vi "AllTogether.vi"() -> ()   [LabVIEW 2022 SP3]
uses:
  <vilib>/DAQmx/read.llb/DAQmx Read (Digital Bool 1Line 1Point).vi
  <vilib>/DAQmx/read.llb/DAQmx Read (Analog 1D DBL NChan 1Samp).vi
  <vilib>/DAQmx/write.llb/DAQmx Write (Digital Bool 1Line 1Point).vi
  <vilib>/DAQmx/create/channels.llb/DAQmx Create Channel (AI-Voltage-Basic).vi
  <vilib>/DAQmx/create/channels.llb/DAQmx Create Channel (DO-Digital Output).vi
  <vilib>/DAQmx/miscellaneous.llb/DAQmx Fill In Error Info.vi
  <vilib>/DAQmx/create/channels.llb/DAQmx Create Channel (DI-Digital Input).vi
panel:
  in  "Numeric 3":dbl
  out "error out":errorcluster
  in  "lines 2":tag
  in  "Connect":bool
  in  "VISA resource name":refnum<visa-resource-name>
  out "connected":bool
  in  "Numeric 2":dbl
  in  "stop 3":bool
  out "Weight Range":dbl(knob) scale=0.0..1500.0
  in  "physical channels":tag
  out "Timer":i32
  out "Numeric":i32
  in  "stop":bool
  out "Buzzer":bool
  in  "lines":tag
  # "Smart Refridgerator System"
  # "Weight Sensor"
  # "Contact Sensor"
  # "Water Level sensor and DC motor control"
  # "g"
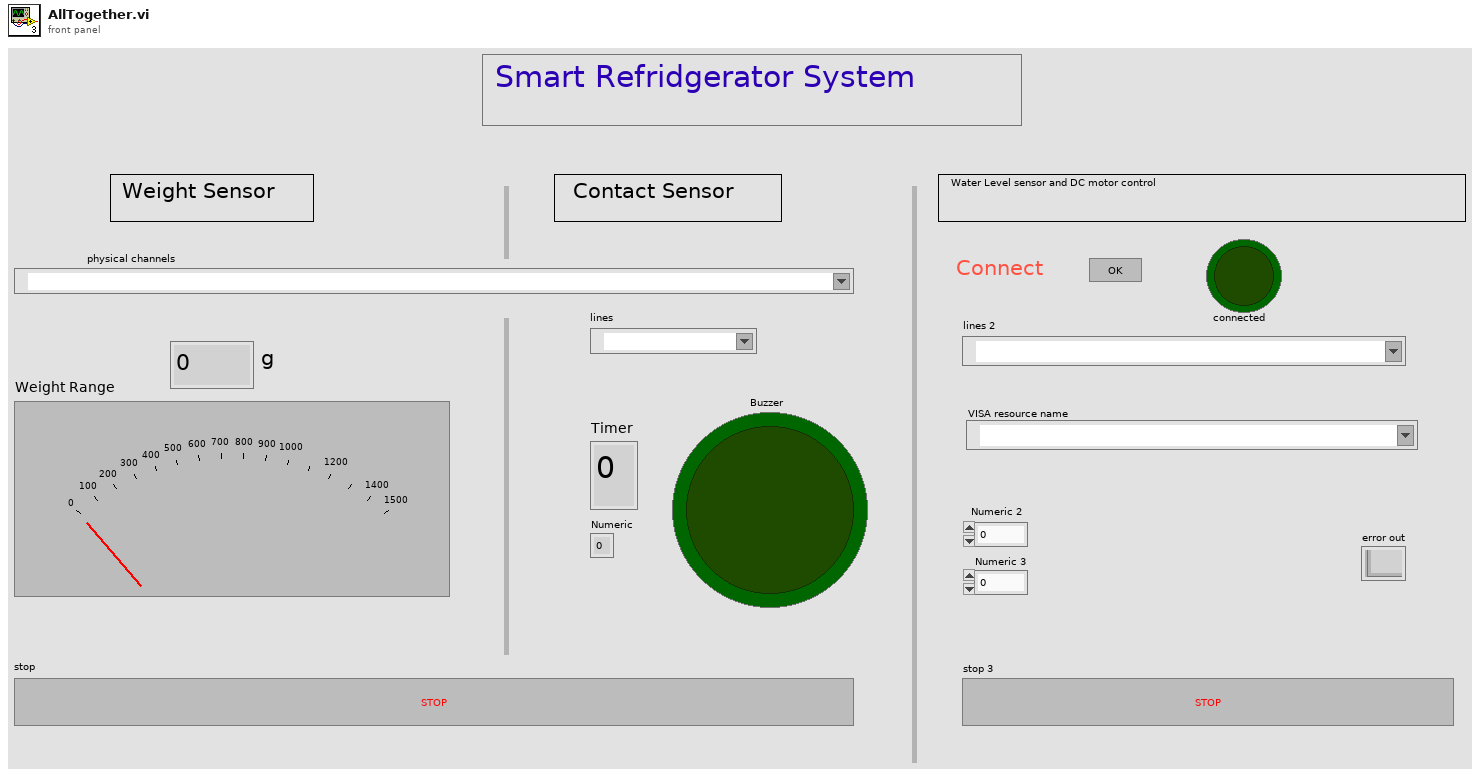
[diagram p1: front panel]
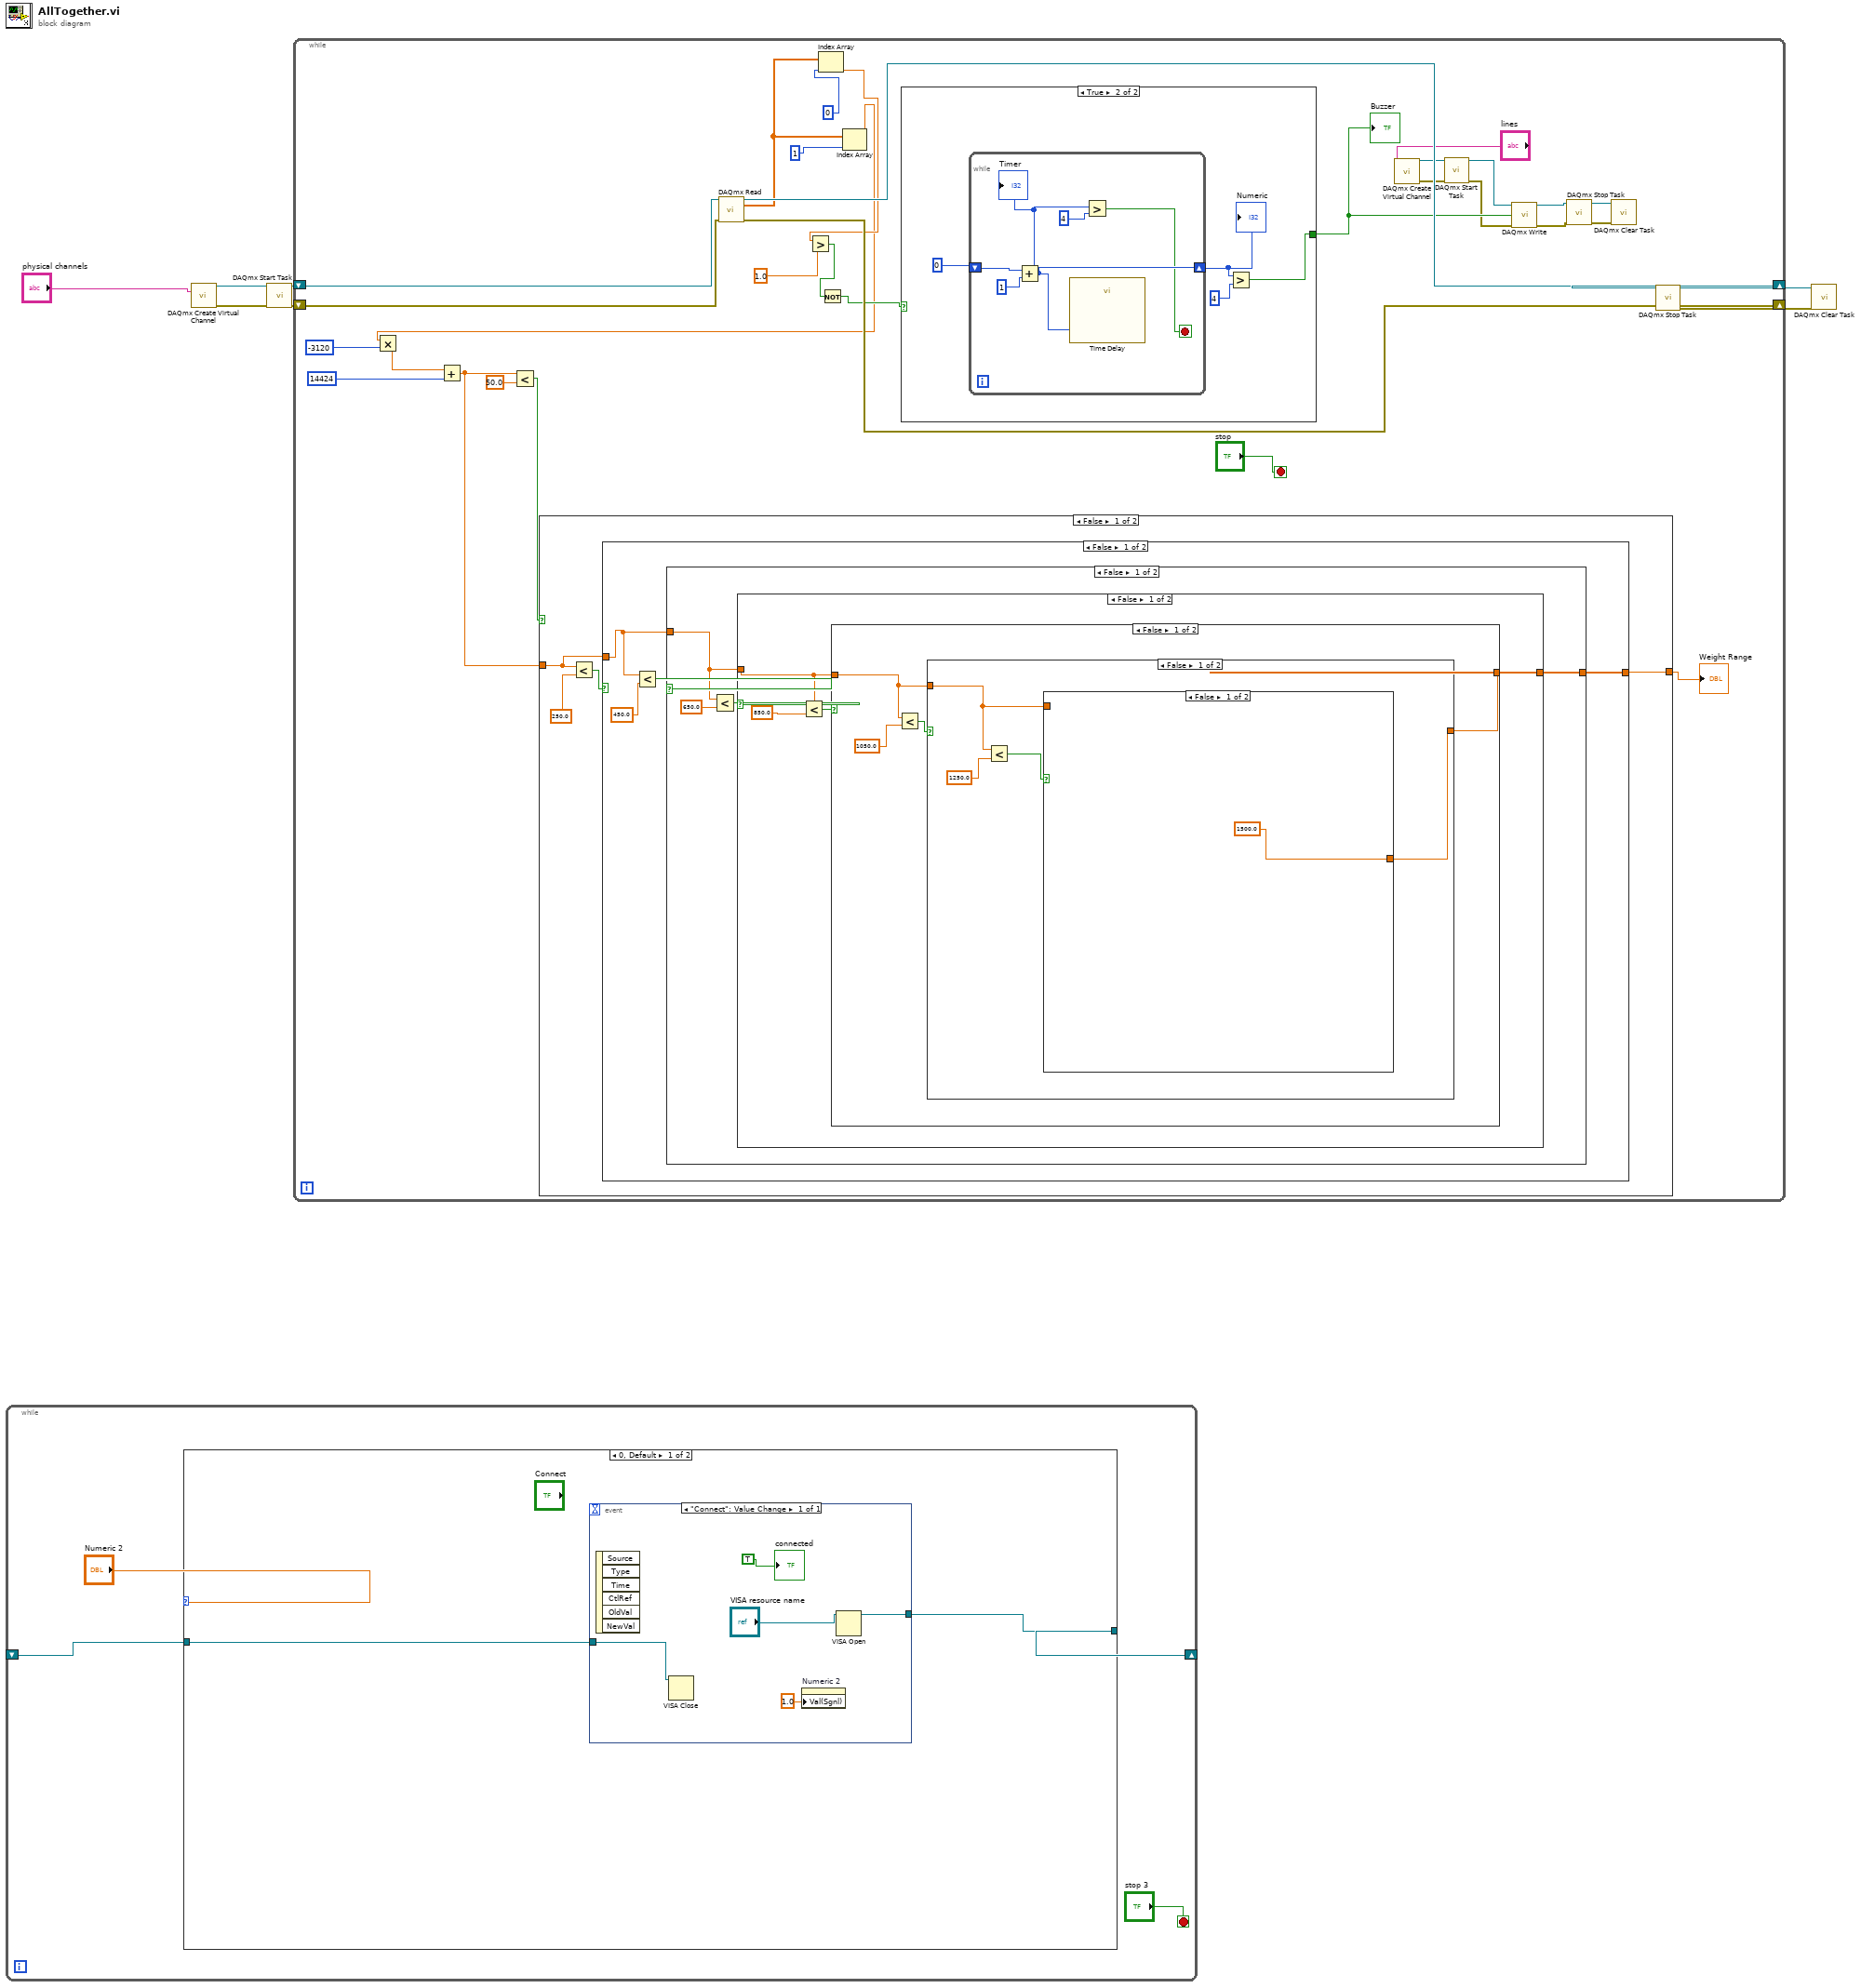
[diagram p0: block diagram]
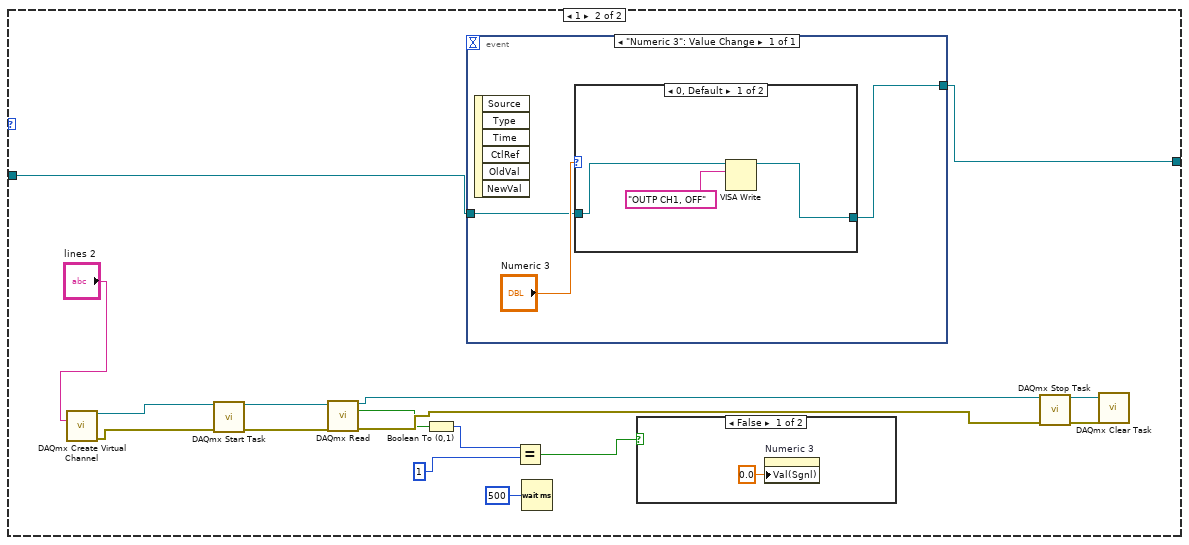
[diagram p2: hidden frame]
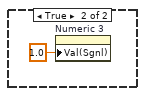
[diagram p3: hidden frame]
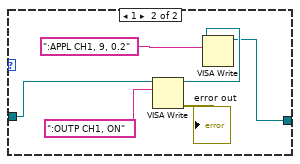
[diagram p4: hidden frame]
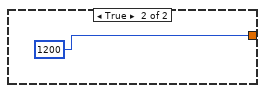
[diagram p5: hidden frame]
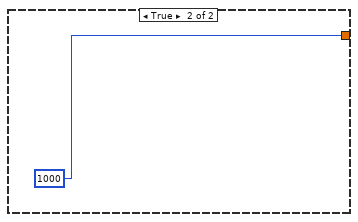
[diagram p6: hidden frame]
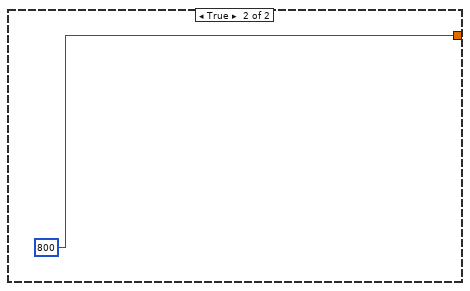
[diagram p7: hidden frame]
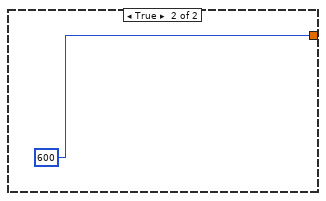
[diagram p8: hidden frame]
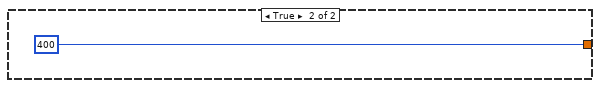
[diagram p9: hidden frame]
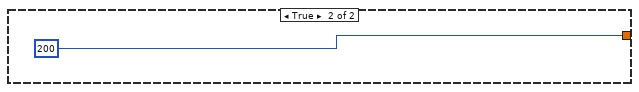
[diagram p10: hidden frame]
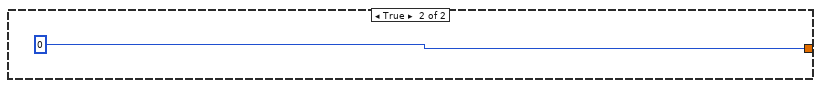
[diagram p11: hidden frame]
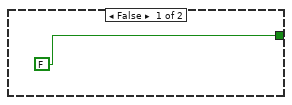
[diagram p12: hidden frame]
diagram:
  n1 = while {
    shift-right: [w13] -> _
    shift-left: _ -> [w11]
    stop <- "stop 3" stop-if-true
    n2 = case shown="0, Default" "Numeric 2" {
      tunnel: [w14 w36] -> w13
      tunnel: w11 -> [w15 w35]
      frame 0, Default {
        n3 = event shown="[0] \"Connect\": Value Change" {
          selector: _ -> [_]
          dyn-events: _ -> [_]
          timeout: _ -> [_]
          tunnel: w15 -> [w20]
          tunnel: [w18] -> w14
          event "Connect": Value Change {
            n4 = event-data() -> ()  [unwired: 1 in, 6 out]
            n5 = VISA Close(VISA resource name=w20) -> ()  [unwired: 1 in, 1 out]
            n6 = property on="Numeric 2" class="DigNum (strict)"("Val(Sgnl)"=1.0 ("Value (Signaling)")) -> ()  [unwired: 2 in, 2 out]
            n7 = VISA Open(VISA resource name="VISA resource name") -> (VISA resource name=w18:refnum<visa-resource-name>)  [unwired: 4 in, 1 out]
            "connected" <- TRUE
          }
        }
      }
      frame 1 {
        n8 = call-poly <vilib>:"DAQmx Create Virtual Channel.vi"("lines"="lines 2") -> ("task out"=w29:refnum<k21>, "error out"=w28:errorcluster)  [unwired: 13 in]
        n9 = call <vilib>:"DAQmx Start Task.vi"("task/channels in"=w29, "error in"=w28) -> ("task out"=w31:refnum<k21>, "error out"=w30:errorcluster)  [unwired: 12 in]
        n10 = call-poly <vilib>:"DAQmx Read.vi"("task/channels in"=w31, "error in"=w30) -> ("task out"=w26:refnum<k21>, "data"=w21:bool, "error out"=w25:errorcluster)  [unwired: 11 in]
        n11 = Boolean To (0,1)(Boolean=w21) -> (0, 1=w33:i16)
        n12 = event shown="[0] \"Numeric 3\": Value Change" {
          selector: _ -> [_]
          dyn-events: _ -> [_]
          timeout: _ -> [_]
          tunnel: [w41] -> w36
          tunnel: w35 -> [w39]
          event "Numeric 3": Value Change {
            n13 = event-data() -> ()  [unwired: 1 in, 6 out]
            n14 = case shown="0, Default" "Numeric 3" {
              tunnel: [w43 w47] -> w41
              tunnel: w39 -> [w42 w46]
              frame 0, Default {
                n15 = VISA Write(VISA resource name=w42, write buffer="OUTP CH1, OFF") -> (VISA resource name out=w43:refnum<visa-resource-name>)  [unwired: 1 in, 2 out]
              }
              frame 1 {
                n16 = VISA Write(VISA resource name=w46, write buffer=":OUTP CH1, ON") -> (VISA resource name out=w48:refnum<visa-resource-name>, error out=→"error out":errorcluster)  [unwired: 1 in, 1 out]
                n17 = VISA Write(VISA resource name=w48, write buffer=":APPL CH1, 9, 0.2") -> (VISA resource name out=w47:refnum<visa-resource-name>)  [unwired: 1 in, 2 out]
              }
            }
          }
        }
        n18 = Equal?(x=w33, y=1) -> (x = y?=w34:bool)
        n19 = Wait (ms)(milliseconds to wait=u32 500) -> ()  [unwired: 1 out]
        n20 = case shown="False" w34 {
          frame False {
            n21 = property on="Numeric 3" class="DigNum (strict)"("Val(Sgnl)"=0.0 ("Value (Signaling)")) -> ()  [unwired: 2 in, 2 out]
          }
          frame True {
            n22 = property on="Numeric 3" class="DigNum (strict)"("Val(Sgnl)"=1.0 ("Value (Signaling)")) -> ()  [unwired: 2 in, 2 out]
          }
        }
        n23 = call <vilib>:"DAQmx Stop Task.vi"("task/channels in"=w26, "error in"=w25) -> ("task out"=w24:refnum<k21>, "error out"=w23:errorcluster)  [unwired: 12 in]
        n24 = call <vilib>:"DAQmx Clear Task.vi"("task in"=w24, "error in"=w23) -> ()  [unwired: 13 in, 1 out]
      }
    }
  }
  n25 = call-poly <vilib>:"DAQmx Create Virtual Channel.vi"("physical channels"="physical channels") -> ("task out"=w9:refnum<k21>, "error out"=w8:errorcluster)  [unwired: 13 in]
  n26 = call <vilib>:"DAQmx Start Task.vi"("task/channels in"=w9, "error in"=w8) -> ("task out"=w7:refnum<k21>, "error out"=w6:errorcluster)  [unwired: 12 in]
  n27 = while {
    shift-right: [w77] -> w3
    shift-left: w7 -> [w79]
    shift-right: [w76] -> w2
    shift-left: w6 -> [w78]
    stop <- "stop" stop-if-true
    n28 = call-poly <vilib>:"DAQmx Read.vi"("task/channels in"=w79, "error in"=w78) -> ("task out"=w77:refnum<k21>, "data"=w52:dbl[], "error out"=w76:errorcluster)  [unwired: 11 in]
    n29 = Index Array(array=w52, index=0) -> (element=w54:dbl)
    n30 = Greater?(x=w54, y=1.0) -> (0:w74:bool)
    n31 = Not(x=w74) -> (.not. x?=w73:bool)
    n32 = Index Array(array=w52, index=1) -> (element=w51:dbl)
    n33 = Multiply(x=w51, y=-3120) -> (x*y=w61:dbl)
    n34 = Add(x=w61, y=14424) -> (x+y=w62:dbl)
    n35 = Less?(x=w62, y=50.0) -> (x < y?=w56:bool)
    n36 = case shown="False" w56 {
      tunnel: [w83 0] -> w57
      tunnel: w62 -> [w82 _]
      frame False {
        n37 = Less?(x=w82, y=250.0) -> (x < y?=w81:bool)
        n38 = case shown="False" w81 {
          tunnel: [w87 200] -> w83
          tunnel: w82 -> [w85 _]
          frame False {
            n39 = Less?(x=w85, y=450.0) -> (x < y?=w86:bool)
            n40 = case shown="False" w86 {
              tunnel: [w89 400] -> w87
              tunnel: w85 -> [w90 _]
              frame False {
                n41 = Less?(x=w90, y=650.0) -> (x < y?=w91:bool)
                n42 = case shown="False" w91 {
                  tunnel: w90 -> [w94 _]
                  tunnel: [w93 600] -> w89
                  frame False {
                    n43 = Less?(x=w94, y=850.0) -> (x < y?=w95:bool)
                    n44 = case shown="False" w95 {
                      tunnel: w94 -> [w98 _]
                      tunnel: [w97 800] -> w93
                      frame False {
                        n45 = Less?(x=w98, y=1050.0) -> (x < y?=w99:bool)
                        n46 = case shown="False" w99 {
                          tunnel: [w101 1000] -> w97
                          tunnel: w98 -> [w102 _]
                          frame False {
                            n47 = Less?(x=w102, y=1250.0) -> (x < y?=w103:bool)
                            n48 = case shown="False" w103 {
                              tunnel: [1500.0 ("y") 1200] -> w101
                              tunnel: w102 -> [_ _]
                              frame False {
                              }
                              frame True {
                              }
                            }
                          }
                          frame True {
                          }
                        }
                      }
                      frame True {
                      }
                    }
                  }
                  frame True {
                  }
                }
              }
              frame True {
              }
            }
          }
          frame True {
          }
        }
      }
      frame True {
      }
    }
    "Weight Range" <- w57
    n49 = case shown="True" w73 {
      tunnel: [FALSE w114] -> w72
      frame False {
      }
      frame True {
        n50 = while {
          shift-right: [w119] -> w117
          shift-left: 0 -> [w122]
          stop <- w118 stop-if-true
          n51 = Add(x=w122, y=1) -> (x+y=w119:i32)
          "Timer" <- w119
          n52 = call "Time Delay"("Delay Time (s)"=w119) -> ()  [unwired: 10 in, 1 out]
          n53 = Greater?(x=w119, y=4) -> (0:w118:bool)
        }
        "Numeric" <- w117
        n54 = Greater?(x=w117, y=4) -> (0:w114:bool)
      }
    }
    "Buzzer" <- w72
    n55 = call-poly <vilib>:"DAQmx Create Virtual Channel.vi"("lines"="lines") -> ("task out"=w70:refnum<k21>, "error out"=w69:errorcluster)  [unwired: 13 in]
    n56 = call <vilib>:"DAQmx Start Task.vi"("task/channels in"=w70, "error in"=w69) -> ("task out"=w68:refnum<k21>, "error out"=w67:errorcluster)  [unwired: 12 in]
    n57 = call-poly <vilib>:"DAQmx Write.vi"("task/channels in"=w68, "data"=w72, "error in"=w67) -> ("task out"=w66:refnum<k21>, "error out"=w65:errorcluster)  [unwired: 10 in, 1 out]
    n58 = call <vilib>:"DAQmx Stop Task.vi"("task/channels in"=w66, "error in"=w65) -> ("task out"=w64:refnum<k21>, "error out"=w63:errorcluster)  [unwired: 12 in]
    n59 = call <vilib>:"DAQmx Clear Task.vi"("task in"=w64, "error in"=w63) -> ()  [unwired: 13 in, 1 out]
  }
  n60 = call <vilib>:"DAQmx Stop Task.vi"("task/channels in"=w3, "error in"=w2) -> ("task out"=w5:refnum<k21>, "error out"=w4:errorcluster)  [unwired: 12 in]
  n61 = call <vilib>:"DAQmx Clear Task.vi"("task in"=w5, "error in"=w4) -> ()  [unwired: 13 in, 1 out]
